vi "HovaCAL_Interface_SetComponentConcentration.vi"(8 "error in (no error)":errorcluster caption="Fehler (Eingang, kein Fehler)", 10 "AutoLin MFV Index":u32, 11 "Konzentration":dbl) -> (0 "error out":errorcluster caption="Fehler (Ausgang)", 2 "AutoLin MFV Index out":u32, 3 "Konzentration out":dbl)   [LabVIEW 2020, in "Linearisierung v2.lvlib" / "Gasteiler.lvlib" / "HovaCAL_Interface.lvlib" / "Kommunikation.lvlib"]
uses:
  Kommunikation.lvlib
  Aktion_FGV_HovaCAL_Interface_GetData.ctl
  Aktion_FGV_HovaCAL_Interface_SetData.ctl
  Aktion_FGV_HovaCAL_Interface_Kommandos.ctl
  Aktion_FGV_HovaCAL_Interface_Kommunikation.ctl
  Controls/Pump Concentration Mode.ctl
  Controls/Controls.lvlib
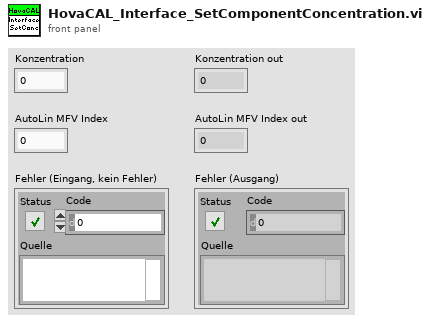
[diagram p1: front panel]
types:
  T1 = typedef "Linearisierung v2.lvlib/Gasteiler.lvlib/HovaCAL_Interface.lvlib/Kommunikation.lvlib/Aktion_FGV_HovaCAL_Interface_GetData.ctl" = enum16{"lesen", "SystemInfo", "MFC Info", "actual Values", "Limits", "first contact"}
  T2 = typedef "Linearisierung v2.lvlib/Gasteiler.lvlib/HovaCAL_Interface.lvlib/Controls.lvlib/Info Cluster.ctl" = cluster{"device":string, "version":string, "number of mfc":i32, "number of pumps":i32, "number of temp controllers":i32, "number of mfs":i32, "number of balances":i32}
  T3 = typedef "Linearisierung v2.lvlib/Gasteiler.lvlib/HovaCAL_Interface.lvlib/Kommunikation.lvlib/Aktion_FGV_HovaCAL_Interface_SetData.ctl" = enum16{"lesen", "Konzentrationen", "Pumpen Parameter", "Pumpe Konzentration", "Pumpe run", "Temperaturen", "Fluss", "Limits", "init"}
  T4 = typedef "Linearisierung v2.lvlib/Gasteiler.lvlib/HovaCAL_Interface.lvlib/Kommunikation.lvlib/Aktion_FGV_HovaCAL_Interface_Kommunikation.ctl" = enum16{"Initialisieren", "Set Konzentrationen", "Set Gase", "Set Limits", "Get Dynamische Werte", "Beenden", "Com ändern", "Get Gase init", "Pause", "Get Gasteiler Infos", "Get MFC Infos", "Set Pumpen Parameter", "Set Pumpe Konzenration", "Set Pumpe run", "Set Temperaturen", "Set Fluss", "Get Gase", "Get Limits", "Get Dynamische Werte 1", "Get Dynamische Werte 2"}
  T5 = typedef "Linearisierung v2.lvlib/Gasteiler.lvlib/HovaCAL_Interface.lvlib/Kommunikation.lvlib/Aktion_FGV_HovaCAL_Interface_Kommandos.ctl" = enum16{"lesen", "verarbeiten", "hinzufügen", "on top", "init", "sammeln", "freigeben", "connected"}
  T6 = cluster{"input concentration setpoint":dbl, "output concentration setpoint":dbl}[]
  T7 = cluster{"input concentration setpoint":dbl, "output concentration setpoint":dbl}
  T8 = typedef "Linearisierung v2.lvlib/Gasteiler.lvlib/HovaCAL_Interface.lvlib/Controls.lvlib/Pump Concentration Mode.ctl" = i32
  T9 = typedef "Linearisierung v2.lvlib/Gasteiler.lvlib/HovaCAL_Interface.lvlib/Controls.lvlib/Reagent.ctl" = i32
  T10 = cluster{"concentratio mode":T8, "Reagent":T9, "Molarity":dbl, "density":dbl, "syringe":dbl, "pump_a":dbl}[]
  T11 = typedef "Linearisierung v2.lvlib/Gasteiler.lvlib/HovaCAL_Interface.lvlib/Controls.lvlib/Pump Concentration.ctl" = cluster{"reagent conc SP":dbl, "water conc SP":dbl}
  T12 = cluster{"concentratio mode":T8, "Reagent":T9, "Molarity":dbl, "density":dbl, "syringe":dbl, "pump_a":dbl}
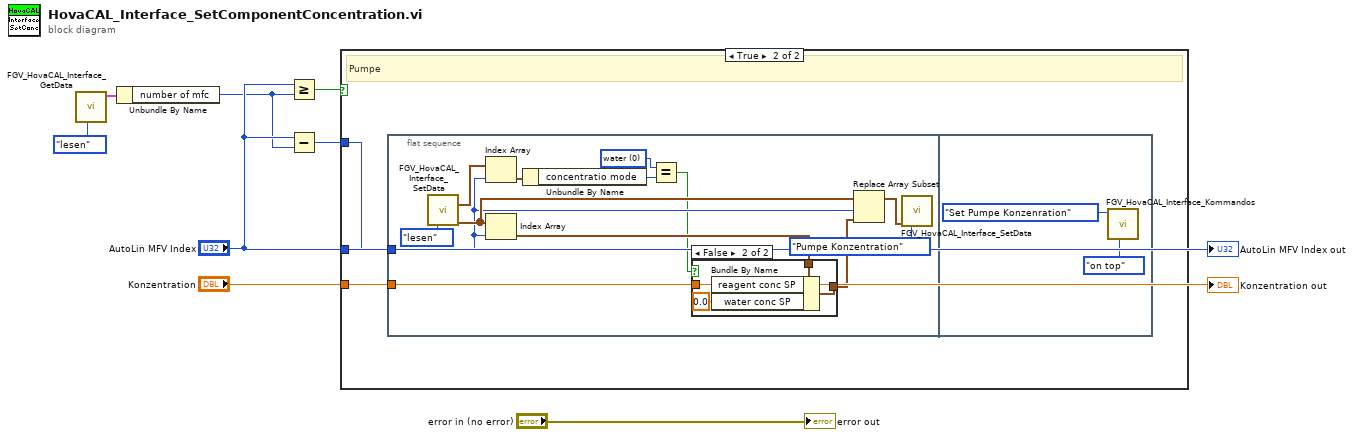
[diagram p0: block diagram]
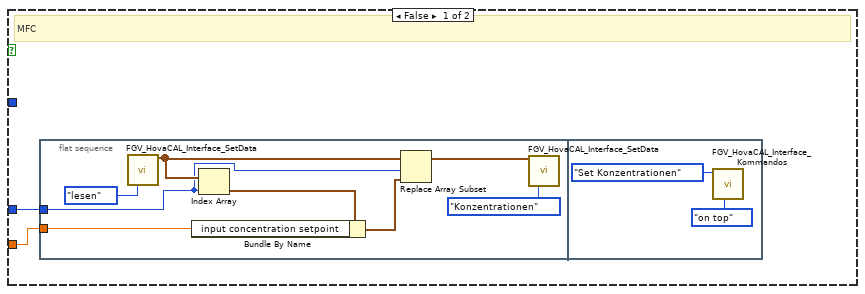
[diagram p2: hidden frame]
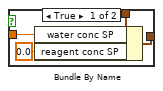
[diagram p3: hidden frame]
diagram:
  n1 = call "FGV_HovaCAL_Interface_GetData.vi"("Aktion"=Aktion_FGV_HovaCAL_Interface_GetData."lesen") -> ("System Cluster out"=w6:T2)  [unwired: 6 in, 4 out]
  n2 = Unbundle By Name(w6) -> ("number of mfc"=w4:i32)
  n3 = Greater Or Equal?(x="AutoLin MFV Index", y=w4) -> (x >= y?=w3:bool)
  n4 = Subtract(x="AutoLin MFV Index", y=w4) -> (x-y=w2:u32)
  n5 = case shown="True" w3 {
    tunnel: "Konzentration" -> [w10 w22]
    tunnel: "AutoLin MFV Index" -> [w9 _]
    tunnel: w2 -> [_ w21]
    frame False {
      # "MFC"
      n6 = flat-sequence {
        tunnel: w9 -> [w15]
        tunnel: w10 -> [w11]
        frame #0 {
          n7 = call "FGV_HovaCAL_Interface_SetData.vi"("Aktion"=Aktion_FGV_HovaCAL_Interface_SetData."lesen") -> ("Set Values Cluster out"=w16:T6)  [unwired: 8 in, 6 out]
          n8 = Index Array(array=w16, index=w15) -> (element=w17:T7)
          n9 = Bundle By Name(cluster=w17, "input concentration setpoint"=w11) -> (w14:T7)
          n10 = Replace Array Subset(array=w16, new element=w14, index=w15) -> (w12:T6)
          n11 = call "FGV_HovaCAL_Interface_SetData.vi"("Set Values Cluster in"=w12, "Aktion"=Aktion_FGV_HovaCAL_Interface_SetData."Konzentrationen") -> ()  [unwired: 7 in, 7 out]
        }
        frame #1 {
          n12 = call "FGV_HovaCAL_Interface_Kommandos.vi"("Aktion"=Aktion_FGV_HovaCAL_Interface_Kommandos."on top", "Kommando in"=Aktion_FGV_HovaCAL_Interface_Kommunikation."Set Konzentrationen") -> ()  [unwired: 3 in, 6 out]
        }
      }
    }
    frame True {
      # "Pumpe"
      n13 = flat-sequence {
        tunnel: w21 -> [w27]
        tunnel: w22 -> [w31]
        frame #0 {
          w24 = T8 0 items=["water", "reagent"] ("x")
          n14 = call "FGV_HovaCAL_Interface_SetData.vi"("Aktion"=Aktion_FGV_HovaCAL_Interface_SetData."lesen") -> ("PumpMode-Cluster out"=w28:T10, "Pump Concentrations-Cluster out"=w30:T11[])  [unwired: 8 in, 5 out]
          n15 = Index Array(array=w28, index=w27) -> (element=w26:T12)
          n16 = Index Array(array=w30, index=w27) -> (element=w34:T11)
          n17 = Unbundle By Name(w26) -> ("concentratio mode"=w25:T8)
          n18 = Equal?(x=w24, y=w25) -> (x = y?=w23:bool)
          n19 = case shown="False" w23 {
            tunnel: w34 -> [w39 w43]
            tunnel: [w38 w42] -> w33
            tunnel: w31 -> [w37 w41]
            frame True {
              n20 = Bundle By Name(cluster=w39, "water conc SP"=w37, "reagent conc SP"=0.0) -> (w38:T11)
            }
            frame False {
              n21 = Bundle By Name(cluster=w43, "reagent conc SP"=w41, "water conc SP"=0.0) -> (w42:T11)
            }
          }
          n22 = Replace Array Subset(array=w30, new element=w33, index=w27) -> (w29:T11[])
          n23 = call "FGV_HovaCAL_Interface_SetData.vi"("Pump Concentrations-Cluster"=w29, "Aktion"=Aktion_FGV_HovaCAL_Interface_SetData."Pumpe Konzentration") -> ()  [unwired: 7 in, 7 out]
        }
        frame #1 {
          n24 = call "FGV_HovaCAL_Interface_Kommandos.vi"("Aktion"=Aktion_FGV_HovaCAL_Interface_Kommandos."on top", "Kommando in"=Aktion_FGV_HovaCAL_Interface_Kommunikation."Set Pumpe Konzenration") -> ()  [unwired: 3 in, 6 out]
        }
      }
    }
  }
  "error out" <- "error in (no error)"
  "AutoLin MFV Index out" <- "AutoLin MFV Index"
  "Konzentration out" <- "Konzentration"
